vi "Append Links to Subdirectories.vi"(0 "high level report in":string, 1 "md path":path, 5 "current path":path, 7 "directories within current path":path[](array[path]), 11 "error in":errorcluster) -> (4 "high level report out":string, 15 "error out":errorcluster)   [LabVIEW 2019, in "MD Generator.lvlib"]
uses:
  MD Generator.lvlib
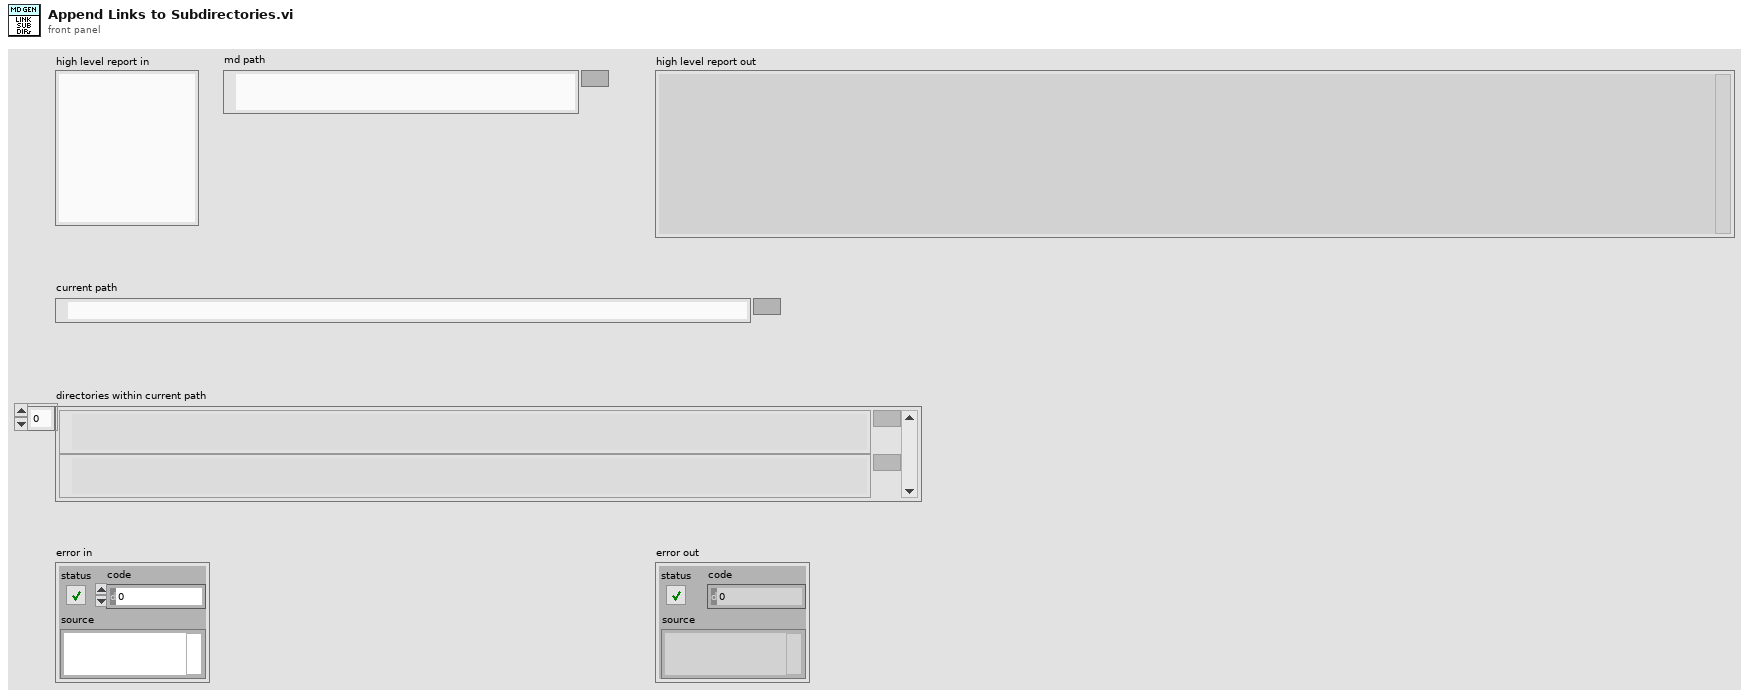
[diagram p1: front panel]
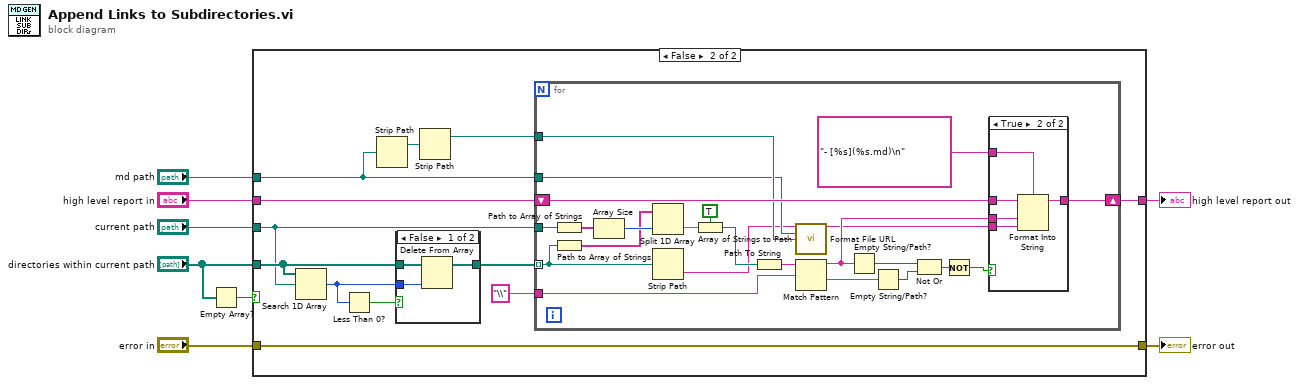
[diagram p0: block diagram]
diagram:
  n1 = Empty Array?(array="directories within current path") -> (empty?=w2:bool)
  n2 = case shown="False" w2 {
    tunnel: [w9 w22] -> w8
    tunnel: "error in" -> [w9 w22]
    tunnel: [w10 w16] -> w6
    tunnel: "high level report in" -> [w10 w17]
    tunnel: "current path" -> [_ w11]
    tunnel: "directories within current path" -> [_ w19]
    tunnel: "md path" -> [_ w15]
    frame True {
    }
    frame False {
      n3 = Search 1D Array(1D array=w19, element=w11) -> (index of element=w20:i32)  [unwired: 1 in]
      n4 = Less Than 0?(x=w20) -> (x < 0?=w21:bool)
      n5 = Strip Path(path=w15) -> (stripped path=w13:path)  [unwired: 1 out]
      n6 = case shown="False" w21 {
        tunnel: [w54 w55] -> w12
        tunnel: w19 -> [w53 w55]
        tunnel: w20 -> [w52 _]
        frame False {
          n7 = Delete From Array(array=w53, index=w52) -> (array with subset deleted=w54:path[])  [unwired: 1 in, 1 out]
        }
        frame True {
        }
      }
      n8 = Strip Path(path=w13) -> (stripped path=w14:path)  [unwired: 1 out]
      n9 = for {
        tunnel: "\\" ("regular expression") -> [w45]
        tunnel: w15 -> [w41]
        tunnel: w14 -> [w42]
        shift-right: [w43] -> w16
        shift-left: w17 -> [w44]
        tunnel: w12 -> [w23] mode=indexing
        tunnel: w11 -> [w40]
        n10 = Path to Array of Strings(0:w40) -> (2:w39:string[])  [unwired: 1 out]
        n11 = Path to Array of Strings(0:w23) -> (2:w37:string[])  [unwired: 1 out]
        n12 = Array Size(array=w39) -> (size(s)=w38:i32)
        n13 = Split 1D Array(array=w37, index=w38) -> (second subarray=w24:string[])  [unwired: 1 out]
        n14 = Strip Path(path=w23) -> (name=w26:string)  [unwired: 1 out]
        n15 = Array of Strings to Path(0:w24, 1:TRUE ("relative")) -> (2:w36:path)
        n16 = Path To String(path=w36) -> (string=w34:string)
        n17 = call "Format File URL.vi"("file name"=w26, "file dir"=w41, "base dir"=w42) -> ("image URL string"=w25:string)  [unwired: 12 in]
        n18 = Match Pattern(string=w34, regular expression=w45) -> (before substring=w29:string, after substring=w33:string)  [unwired: 1 in, 2 out]
        n19 = Empty String/Path?(string/path=w29) -> (empty?=w31:bool)
        n20 = Empty String/Path?(string/path=w33) -> (empty?=w32:bool)
        n21 = Not Or(1:w32, 2:w31) -> (0:w30:bool)
        n22 = Not(x=w30) -> (.not. x?=w28:bool)
        n23 = case shown="True" w28 {
          tunnel: w44 -> [w46 w51]
          tunnel: [w46 w50] -> w43
          tunnel: w29 -> [_ w49]
          tunnel: "- [%s](%s.md)\n" ("format string") -> [_ w48]
          tunnel: w25 -> [_ w47]
          frame False {
          }
          frame True {
            n24 = Format Into String(format string=w48, initial string=w51, w49, w47) -> (resulting string=w50:string)  [unwired: 1 in, 1 out]
          }
        }
      }
    }
  }
  "error out" <- w8
  "high level report out" <- w6
